vi "WaveFormGraphBuffer.vi"(8 "clear first (no:F)":bool, 9 "chart length (points)":i32=100, 11 "NewPoint":dbl) -> (3 "Value":dbl[](array[numeric]))   [LabVIEW 2023]
doc: "This reentrant VI uses an XY graph to mimic the behavior of an XY chart, in that it plots a stipulated amount of the most recently acquired data points. The chart data is stored in a static local variable of the output XY chart indicator.\n\nBecause the VI has been marked reentrant (in VI setup), you can make multiple parallel calls to the VI without confusing the memory. Use the new points array input to supply multiple points at once, or leave the array unwired (empty) and use the new point cluster input to supply one point at a time. If the locally stored chart array is not equal to chart length, it is expanded to that lenght by replicating the most recently acquired point. Data in excess of the history length is discarded. Set clear first to clear the chart history before processing the new points."
panel:
  in  "Case Constant\n(See Context Help)":bool=TRUE
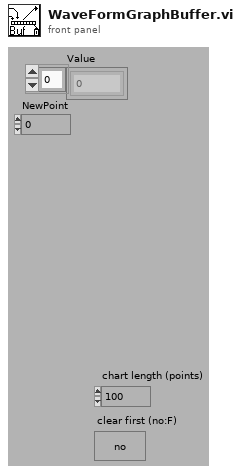
[diagram p1: front panel]
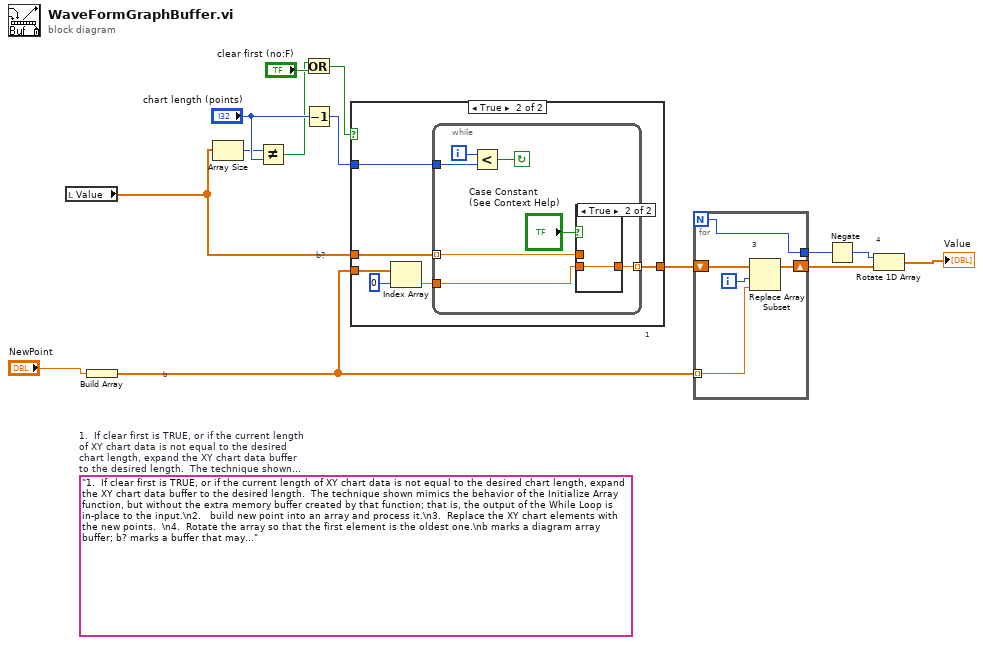
[diagram p0: block diagram]
diagram:
  (unwired) "1.  If clear first is TRUE, or if the current length of XY chart data is not equal to the desired chart length, expand the XY chart data buffer to the desired length.  The technique shown mimics the behavior of the Initialize Array function, but without the extra memory buffer created by that function; that is, the output of the While Loop is in-place to the input.\n2.   build new point into an array and process it.\n3.  Replace the XY chart elements with the new points.  \n4.  Rotate the array so that the first element is the oldest one.\nb marks a diagram array buffer; b? marks a buffer that may be in the calling VI. \n\nModified for waveform by KM"  # 1.  If clear first is TRUE, or if the current length of XY chart data is not equal to the desired chart length, expand the XY chart data buffer to the desired length.  The technique shown mimics the behavior of the Initialize Array function, but without the extra memory buffer created by that function; that is, the output of the While Loop is in-place to the input. 2.   build new point into an array and process it. 3.  Replace the XY chart elements with the new points.   4.  Rotate the array so that the first element is the oldest one. b marks a diagram array buffer; b? marks a buffer that may be in the calling VI.   Modified for waveform by KM
  # "4"
  # "1"
  # "b"
  # "b?"
  n1 = local read "Value"() -> (w3:dbl[])
  n2 = Build Array("NewPoint") -> (w4:dbl[])
  n3 = Array Size(array=w3) -> (size(s)=w10:i32)
  n4 = Not Equal?(x=w10, y="chart length (points)") -> (x != y?=w7:bool)
  n5 = Or(x=w7, y="clear first (no:F)") -> (x .or. y?=w6:bool)
  n6 = Decrement(x="chart length (points)") -> (x-1=w5:i32)
  n7 = case shown="True" w6 {
    tunnel: [w15 w16] -> w11
    tunnel: w5 -> [_ w20]
    tunnel: w3 -> [w15 w21]
    tunnel: w4 -> [_ w18]
    frame False {
    }
    frame True {
      n8 = Index Array(array=w18, index=0) -> (element=w17:dbl)
      n9 = while {
        tunnel: [w24] -> w16 mode=indexing
        tunnel: w17 -> [w22]
        tunnel: w20 -> [w28]
        tunnel: w21 -> [w23] mode=indexing
        i -> [w27]
        stop <- w26 continue-if-true
        n10 = Less?(x=w27, y=w28) -> (x < y?=w26:bool)
        n11 = case shown="True" "Case Constant\n(See Context Help)" {
          tunnel: [w29 w30] -> w24
          tunnel: w23 -> [w29 _]
          tunnel: w22 -> [_ w30]
          frame False {
          }
          frame True {
          }
        }
      }
    }
  }
  n12 = for {
    N -> [w31]
    shift-right: [w35] -> w13
    shift-left: w11 -> [w32]
    tunnel: w4 -> [w33] mode=indexing
    tunnel: [w31] -> w9
    i -> [w34]
    # "3"
    n13 = Replace Array Subset(array=w32, new element=w33, index=w34) -> (w35:dbl[])
  }
  n14 = Negate(x=w9) -> (-x=w14:i32)
  n15 = Rotate 1D Array(1:w13, 2:w14) -> (0:→"Value":dbl[])
